vi "Read Mock Configurable Process.vi"(11 "Configuration File Process Interface Test in":refnum<class "Configuration File Process Interface Test.lvclass">) -> (2 "Mock Configurable.lvclass":refnum<class "Mock Configurable Process.lvclass">, 3 "Configuration File Process Interface Test out":refnum<class "Configuration File Process Interface Test.lvclass">)   [LabVIEW 2020, in "Configuration File Process Interface Test.lvclass"]
uses:
  Configuration File Process Interface Test.lvclass
  Mock Configurable Process/Mock Configurable Process.lvclass
  C:/Git/astemes-triarc-framework/tests/Configuration Interface Test/Configuration Interface Test.lvclass
  Configuration Interface Test/Configuration Interface Test.lvclass
panel:
  out "error out":errorcluster
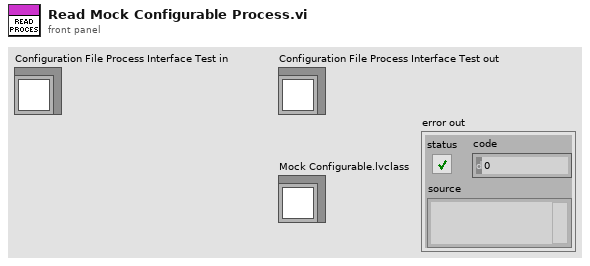
[diagram p1: front panel]
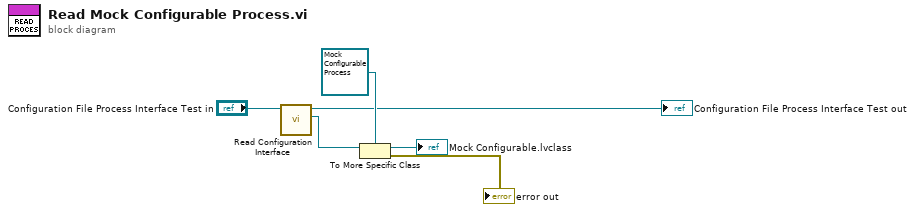
[diagram p0: block diagram]
diagram:
  n1 = call "Read Configuration Interface.vi"("Configuration Interface Test In"="Configuration File Process Interface Test in") -> ("Configuration"=w4:refnum<class "Configuration.lvclass">, "Configuration Interface Test Out"=→"Configuration File Process Interface Test out":refnum<class "Configuration File Process Interface Test.lvclass">)  [unwired: 9 in]
  n2 = To More Specific Class(target class=refnum<class "Mock Configurable Process.lvclass"> refnum ("Mock Configurable.lvclass"), reference=w4) -> (specific class reference=→"Mock Configurable.lvclass":refnum<class "Mock Configurable Process.lvclass">, error out=→"error out":errorcluster)  [unwired: 1 in]
